vi "MQTT_SubAck_Read.vi"(8 "error in (no error)":errorcluster, 11 "SSL_Connection":T2) -> (0 "error out":errorcluster, 1 "Granted QoS Levels":T1[](array[typedef]), 3 "SSL_Connection 2":T2)   [LabVIEW 2018, in "AWS_IoT.lvlib"]
doc: "© 2015 - daq.io, LLC - Peter Adelhardt"
uses:
  AWS_IoT.lvlib
  Controls/SSL_Connection.ctl
  Controls/QoS.ctl
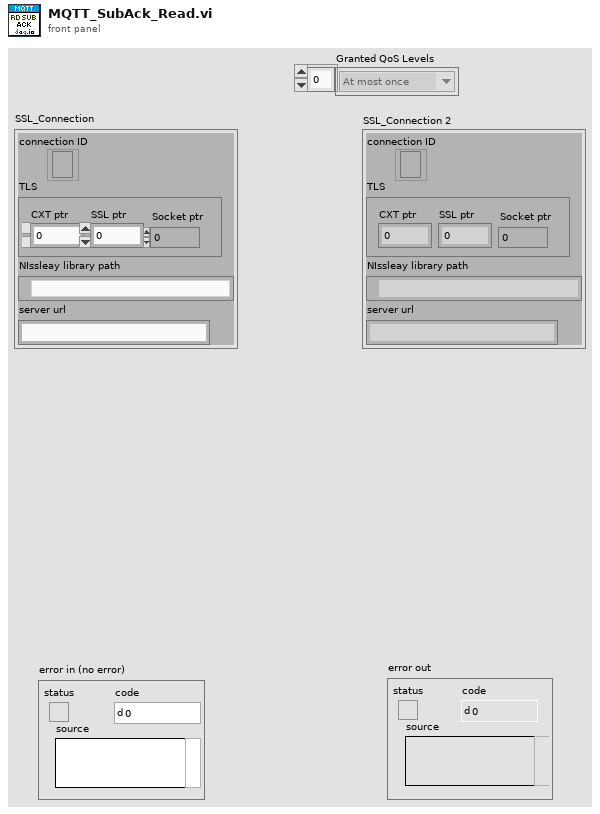
[diagram p1: front panel]
types:
  T1 = typedef "AWS_IoT.lvlib/QoS.ctl" = enum8{"At most once", "At least once", "Exactly once", "Reserved"}
  T2 = typedef "AWS_IoT.lvlib/SSL_Connection.ctl" = cluster{"connection ID":refnum<k5>, "TLS":cluster{"CXT ptr":i32, "SSL ptr":i32, "Socket ptr":i32}, "NIssleay library path":path, "server url":string}
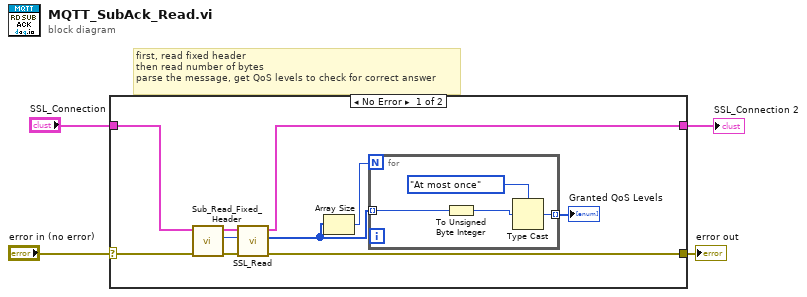
[diagram p0: block diagram]
diagram:
  # "first, read fixed header\nthen read number of bytes\nparse the message, get QoS levels to check for correct answer"
  n1 = case shown="No Error" "error in (no error)" {
    selector: "error in (no error)" -> [w12 w20]
    tunnel: [w10 w20] -> w3
    tunnel: "SSL_Connection" -> [w6 w19]
    tunnel: [w5 w19] -> w1
    frame No Error {
      n2 = call "Sub_Read_Fixed_Header.vi"("error in (no error)"=w12, "SSL_Connection"=w6) -> ("error out"=w11:errorcluster, "Remaining Length"=w13:u32, "SSL_Connection"=w9:T2)  [unwired: 3 in, 4 out]
      n3 = call "SSL_Read.vi"("error in (no error)"=w11, "bytes to read"=w13, "SSL_Connection"=w9) -> ("error out"=w10:errorcluster, "data out"=w8:u8[], "SSL_Connection"=w5:T2)  [unwired: 5 in, 1 out]
      n4 = Array Size(array=w8) -> (size(s)=w14:i32)
      n5 = for {
        N: w14 -> [_]
        tunnel: [w17] -> w7 mode=indexing
        tunnel: w8 -> [w16] mode=indexing
        n6 = To Unsigned Byte Integer(number=w16) -> (unsigned 8bit integer=w15:u8)
        n7 = Type Cast(type=QoS."At most once" ("QoS Level"), x=w15) -> (*(type *) &x=w17:T1)
      }
      "Granted QoS Levels" <- w7
    }
    frame Error {
    }
  }
  "error out" <- w3
  "SSL_Connection 2" <- w1
